vi "LcWebView_AlertDialog_Custom A message with a custom image.vi"() -> ()   [LabVIEW 2018, in "LcWebView.lvclass"]
uses:
  LcWebView.lvclass
  C:/Projects/LcWebView2/LcWebView/LcWebView_class/data/Microsoft.Web.WebView2.WinForms.dll
  data/Microsoft.Web.WebView2.WinForms.dll
  webui/ctrls/DialogWithImage.ctl
panel:
  out "BrowserProcessId":u32
  in  "stop":bool
  out "Result":string
  out "Status Message":string
  in  "Web":refnum<k24>(container)
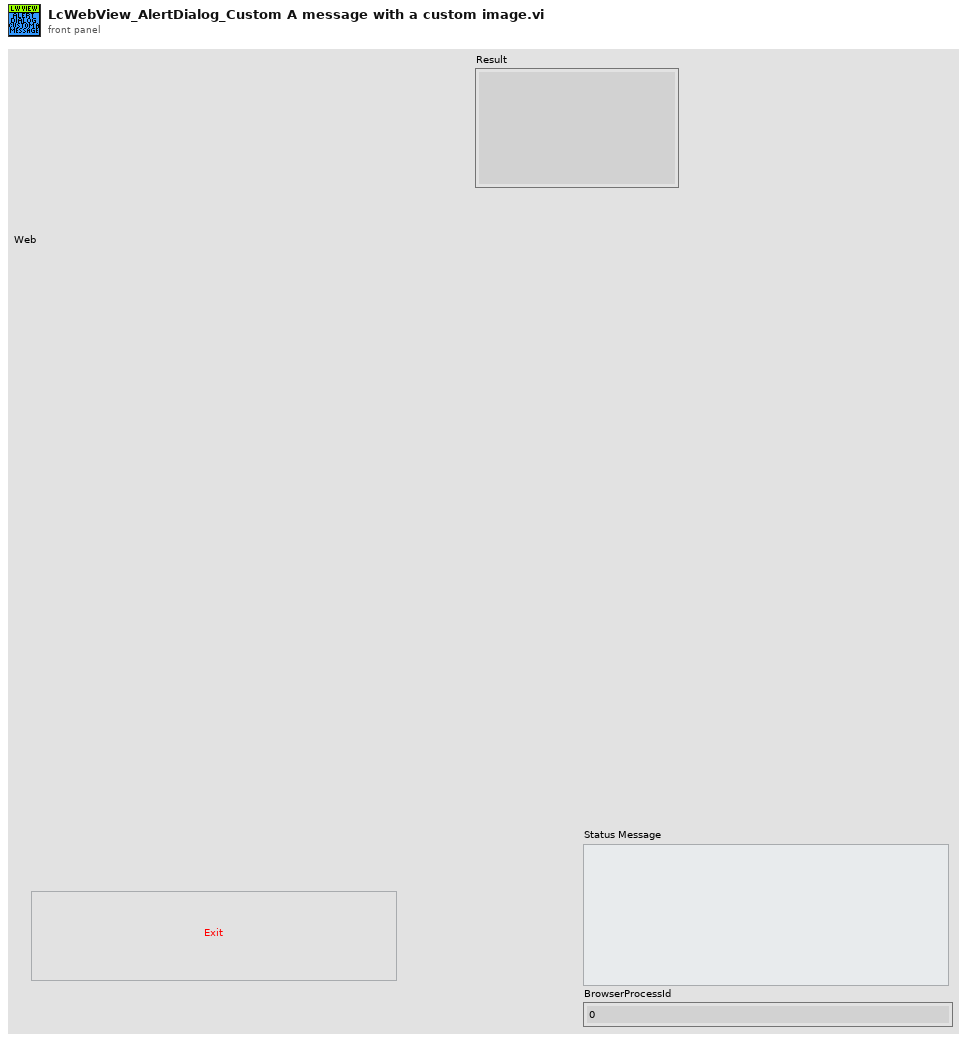
[diagram p1: front panel]
types:
  T1 = typedef "LcWebView.lvclass/DialogWithImage.ctl" = cluster{"title":string, "text":string, "imageUrl":string, "imageAlt":string, "imageWidth":dbl, "imageHeight":dbl}
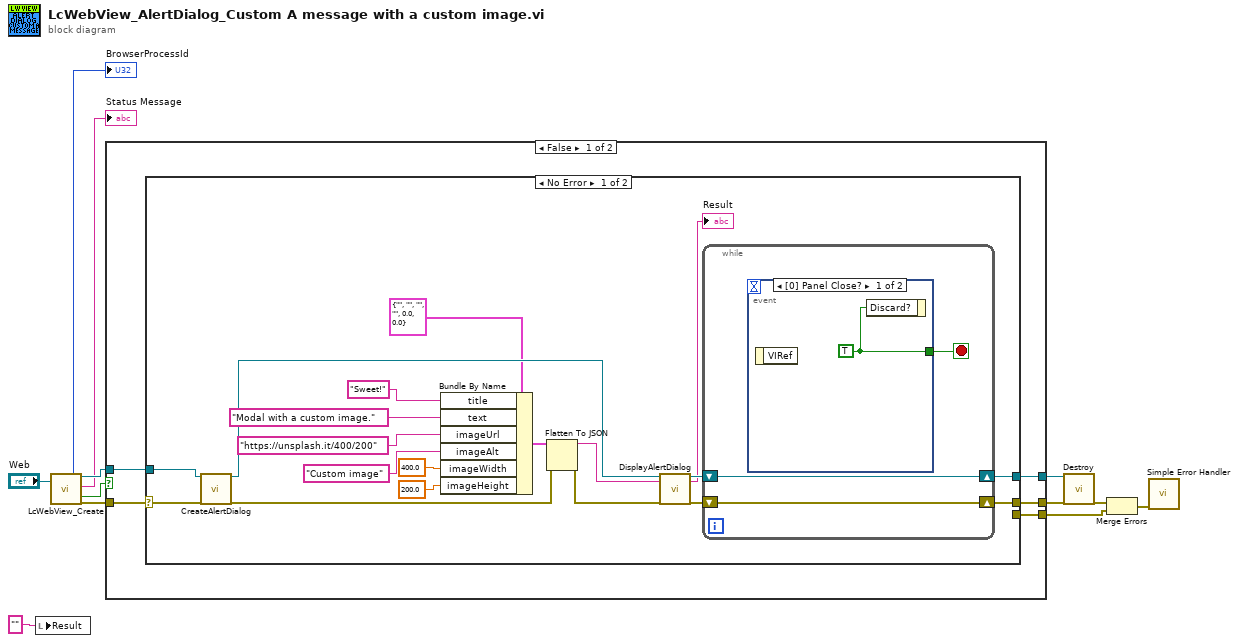
[diagram p0: block diagram]
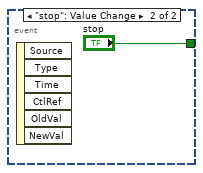
[diagram p2: hidden frame]
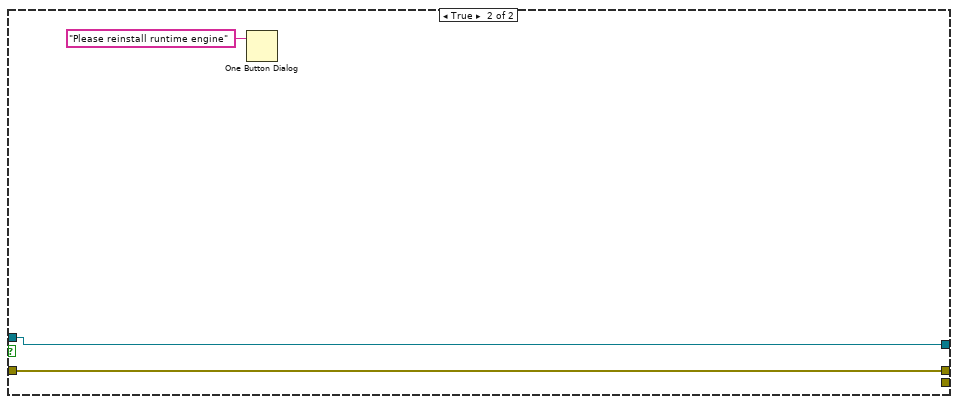
[diagram p4: hidden frame]
diagram:
  n1 = local write "Result"("" ("Result")) -> ()
  n2 = call "LcWebView_Create.vi"("Webview container"="Web") -> ("BrowserProcessId"=→"BrowserProcessId":u32, "reference out"=w11:refnum<class "LcWebView.lvclass">, "Status Message"=→"Status Message":string, "Reinstall Runtime"=w4:bool, "Error Out"=w10:errorcluster)  [unwired: 11 in, 3 out]
  n3 = case shown="False" w4 {
    tunnel: w11 -> [w17 w46]
    tunnel: w10 -> [w16 w45]
    tunnel: [w15 w46] -> w9
    tunnel: [w13 w45] -> w8
    tunnel: [w14 _] -> w5
    frame False {
      n4 = case shown="No Error" w16 {
        selector: w16 -> [w33 w42]
        tunnel: w17 -> [w34 w43]
        tunnel: [w35 w43] -> w15
        tunnel: [w36 _] -> w13
        tunnel: [_ w42] -> w14
        frame No Error {
          n5 = call-dynamic "CreateAlertDialog.vi"("reference in"=w34, "Error In"=w33) -> ("reference out"=w32:refnum<class "LcWebView.lvclass">, "Error Out"=w19:errorcluster)  [unwired: 16 in]
          n6 = Bundle By Name(cluster=T1 {"title"="", "text"="", "imageUrl"="", "imageAlt"="", "imageWidth"=0.0, "imageHeight"=0.0}, "title"="Sweet!", "text"="Modal with a custom image.", "imageUrl"="https://unsplash.it/400/200", "imageAlt"="Custom image", "imageWidth"=400.0, "imageHeight"=200.0) -> (w21:T1)
          n7 = Flatten To JSON(anything=w21, error in (no error)=w19) -> (JSON string=w20:string, 11:w18:errorcluster)  [unwired: 1 in]
          n8 = call-dynamic "DisplayAlertDialog.vi"("reference in"=w32, "Arguments as Json Text"=w20, "Error In"=w18) -> ("reference out"=w31:refnum<class "LcWebView.lvclass">, "Result"=→"Result":string, "Error Out"=w30:errorcluster)  [unwired: 14 in]
          n9 = while {
            shift-right: [w39] -> w35
            shift-left: w31 -> [w39]
            shift-right: [w38] -> w36
            shift-left: w30 -> [w38]
            stop <- w37 stop-if-true
            n10 = event shown="[0] Panel Close?" {
              selector: _ -> [_ _]
              dyn-events: _ -> [_ _]
              timeout: _ -> [_ _]
              tunnel: [w40 "stop"] -> w37
              event Panel Close? {
                w40 = TRUE ("Discard?")
                n11 = event-data() -> ()  [unwired: 1 in, 1 out]
                n12 = event-data("Discard?"=w40) -> ()  [unwired: 1 in, 1 out]
              }
              event "stop": Value Change {
                n13 = event-data() -> ()  [unwired: 1 in, 6 out]
              }
            }
          }
        }
        frame Error {
        }
      }
    }
    frame True {
      n14 = One Button Dialog(message="Please reinstall runtime engine") -> ()  [unwired: 1 in, 1 out]
    }
  }
  n15 = call-dynamic "Destroy.vi"("reference in"=w9, "Error In"=w8) -> ("Error Out"=w7:errorcluster)  [unwired: 16 in, 1 out]
  n16 = Merge Errors(w7, w5) -> (w2:errorcluster)
  n17 = call <vilib>:"Simple Error Handler.vi"("error in (no error)"=w2) -> ()  [unwired: 4 in, 5 out]
